vi "Test PLL.vi"(8 "error in (no error)":errorcluster, 11 "LockinDAQ in":refnum<class "LockinDAQ.lvclass">) -> (0 "error out":errorcluster, 3 "LockinDAQ out":refnum<class "LockinDAQ.lvclass">)   [LabVIEW 2016, in "LockinDAQ.lvclass"]
uses:
  LockinDAQ.lvclass
  Typedefs/AO-cluster.ctl
  Typedefs/Function-enum.ctl
  Typedefs/REF-cluster.ctl
  Typedefs/Sampling.ctl
  LockinDAQ.lvclass/LockinDAQ.ctl
panel:
  out "Waveform Graph":waveform(dbl)[](graph)=[{"t0"=timestamp(0 s since 1904-01-01), "dt"=0.001, "Y"=array[1000 elements]}, {"t0"=timestamp(0 s since 1904-01-01), "dt"=0.001, "Y"=array[1000 elements]}]
  in  "sampling":T1={"Fs"=204789.0, "#s"=15753}
  in  "stop":bool
  out "Channels: Lockin":T2={"Ch"=[1], " f (Hz)"=[13.0], "Phase (°)"=[0.0], "TC (s)"=[0.1], "order"=[1]} {"order" min=1; "TC (s)" min=0.0001 format="%#_3p"; "Phase (°)" format="%.3g"; "f (Hz)" format="%.3g"}
  in  "AO Chanels":T3={"Ch"=[0], "Amp (V)"=[0.01], "DC (V)"=[0.0], "f (Hz)"=[13.0], "Phase (°)"=[0.0], "Function"=[enum."Sine"], "Sweep?"=[FALSE]} {"f (Hz)" min=0.001 max=10000.0 format="%.3g"; "Phase (°)" format="%.3g"; "DC (V)" format="%.3p"; "Amp (V)" min=0.0 max=10.0 format="%.3p"}
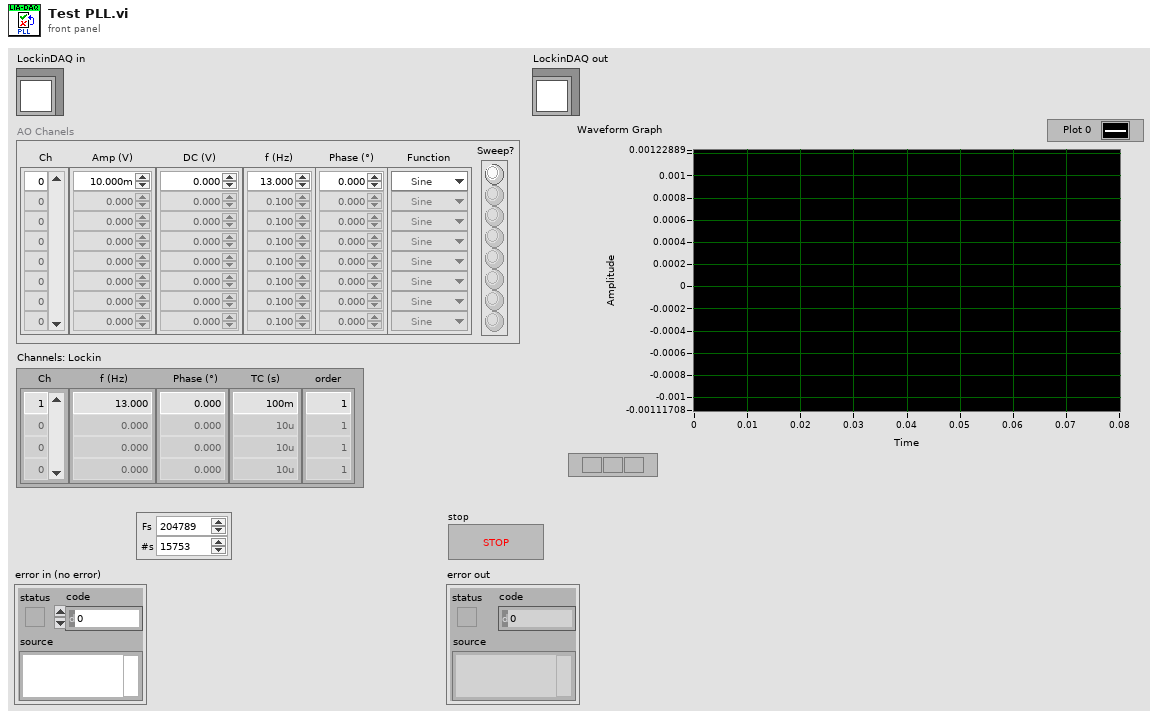
[diagram p1: front panel]
types:
  T1 = typedef "LockinDAQ.lvclass/Sampling.ctl" = cluster{"Fs":dbl, "#s":i32}
  T2 = typedef "LockinDAQ.lvclass/REF-cluster.ctl" = cluster{"Ch":i32[], " f (Hz)":dbl[], "Phase (°)":dbl[], "TC (s)":dbl[], "order":i32[]}
  T3 = typedef "LockinDAQ.lvclass/AO-cluster.ctl" = cluster{"Ch":i32[], "Amp (V)":dbl[], "DC (V)":dbl[], "f (Hz)":dbl[], "Phase (°)":dbl[], "Function":T4[], "Sweep?":bool[]}
  T4 = typedef "LockinDAQ.lvclass/Function-enum.ctl" = enum16{"Sine", "Triangle", "Square", "Sawtooth"}
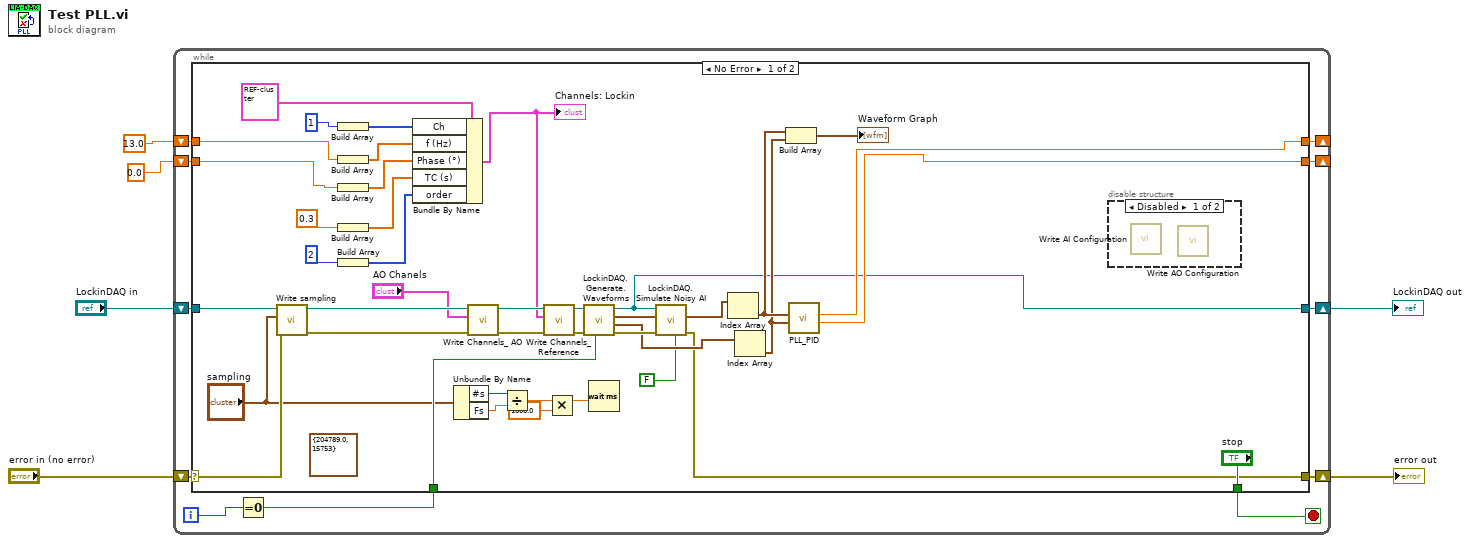
[diagram p0: block diagram]
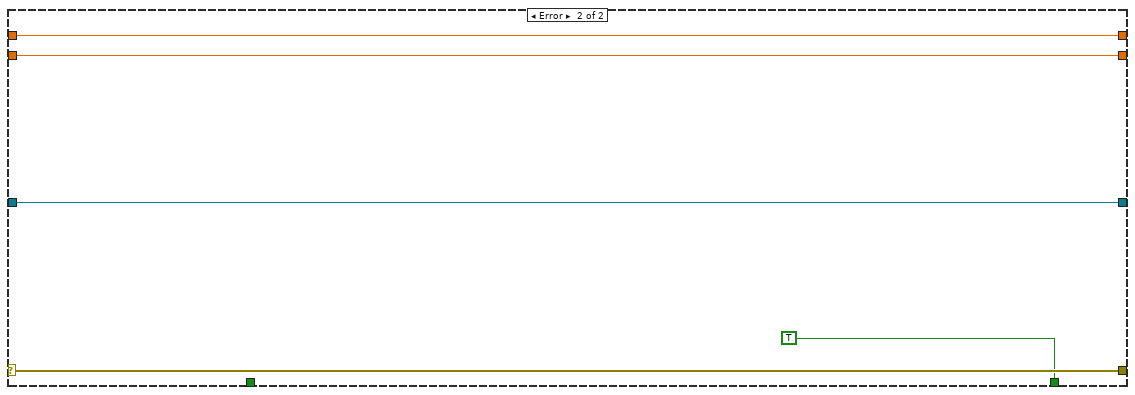
[diagram p3: hidden frame]
diagram:
  n1 = while {
    shift-right: [w16] -> w5
    shift-left: "error in (no error)" -> [w17]
    shift-right: [w14] -> w3
    shift-left: "LockinDAQ in" -> [w15]
    shift-right: [w10] -> _
    shift-left: 13.0 -> [w8]
    shift-right: [w9] -> _
    shift-left: 0.0 -> [w7]
    i -> [w12]
    stop <- w11 stop-if-true
    n2 = Equal To 0?(x=w12) -> (x = 0?=w13:bool)
    n3 = case shown="No Error" w17 {
      selector: w17 -> [w57 w63]
      tunnel: [w18 w63] -> w16
      tunnel: [w24 w62] -> w14
      tunnel: w15 -> [w58 w62]
      tunnel: w13 -> [w51 _]
      tunnel: ["stop" TRUE ("stop")] -> w11
      tunnel: [w37 w59] -> w10
      tunnel: [w36 w60] -> w9
      tunnel: w8 -> [w35 w59]
      tunnel: w7 -> [w34 w60]
      frame No Error {
        (unwired) T1 {"Fs"=204789.0, "#s"=15753} ("sampling")
        n4 = call "Write sampling.vi"("error in (no error)"=w57, "sampling"="sampling", "LockinDAQ"=w58) -> ("error out"=w53:errorcluster, "LockinDAQ out"=w54:refnum<class "LockinDAQ.lvclass">)  [unwired: 7 in]
        n5 = Build Array(1) -> (w39:i32[])
        n6 = Build Array(w35) -> (w40:dbl[])
        n7 = Build Array(w34) -> (w41:dbl[])
        n8 = Build Array(0.3) -> (w42:dbl[])
        n9 = Build Array(2) -> (w43:i32[])
        n10 = Bundle By Name(cluster=T2 {"Ch"=[1], " f (Hz)"=[13.0], "Phase (°)"=[0.0], "TC (s)"=[0.3], "order"=[1]} ("Channels: Lockin"), "Ch"=w39, "f (Hz)"=w40, "Phase (°)"=w41, "TC (s)"=w42, "order"=w43) -> (w38:T2)
        "Channels: Lockin" <- w38
        n11 = Unbundle By Name("sampling") -> ("#s"=w29:i32, "Fs"=w28:dbl)
        n12 = call "Write Channels_ AO.vi"("error in (no error)"=w53, "Channels: AO"="AO Chanels", "LockinDAQ"=w54) -> ("error out"=w55:errorcluster, "LockinDAQ out"=w56:refnum<class "LockinDAQ.lvclass">)  [unwired: 7 in]
        n13 = Divide(x=w29, y=w28) -> (x/y=w27:dbl)
        n14 = call "Write Channels_ Reference.vi"("error in (no error)"=w55, "Channels: Lockin"=w38, "LockinDAQ"=w56) -> ("error out"=w50:errorcluster, "LockinDAQ out"=w49:refnum<class "LockinDAQ.lvclass">)  [unwired: 7 in]
        n15 = Multiply(x=w27, y=1000.0) -> (x*y=w26:dbl)
        n16 = call "LockinDAQ.Generate.Waveforms.vi"("Reset?"=w51, "error in (no error)"=w50, "LockinDAQ"=w49) -> ("error out"=w22:errorcluster, "REF []"=w21:waveform(dbl)[], "AO []"=w23:waveform(dbl)[], "LockinDAQ out"=w24:refnum<class "LockinDAQ.lvclass">)  [unwired: 5 in]
        n17 = Wait (ms)(milliseconds to wait=w26) -> ()  [unwired: 1 out]
        n18 = call "LockinDAQ.Simulate Noisy AI.vi"("Simulate Waveguide [T]"=FALSE, "error in (no error)"=w22, "AO []"=w23, "LockinDAQ"=w24) -> ("error out"=w18:errorcluster, "Noisy AI []"=w20:waveform(dbl)[])  [unwired: 5 in, 1 out]
        n19 = Index Array(array=w20) -> (element=w32:waveform(dbl))  [unwired: 1 in]
        n20 = Index Array(array=w21) -> (element=w31:waveform(dbl))  [unwired: 1 in]
        n21 = Build Array(w32, w31) -> (→"Waveform Graph":waveform(dbl)[])
        n22 = call "PLL_PID.vi"("REF []"=w31, "AO []"=w32) -> ("phase output"=w36:dbl, "frequency output"=w37:dbl)  [unwired: 8 in]
        n23 = disable-structure shown="Disabled" {
          frame Disabled {
            n24 = call "Write AI Configuration.vi"() -> ()  [unwired: 10 in, 2 out]
            n25 = call "Write AO Configuration.vi"() -> ()  [unwired: 10 in, 2 out]
          }
          frame Enabled {
          }
        }
      }
      frame Error {
      }
    }
  }
  "error out" <- w5
  "LockinDAQ out" <- w3
